vi "Dynamixel Single Function.vi"(6 "data":u32, 7 "Function":T1, 10 "dynamixel_id":u8=1, 11 "Com port":refnum<visa-resource-name> caption="instrument handle") -> (0 "error out":errorcluster, 1 "function return":i32)   [LabVIEW 2022 SP3]
uses:
  Sub Vis/Dynamixel Commands.ctl
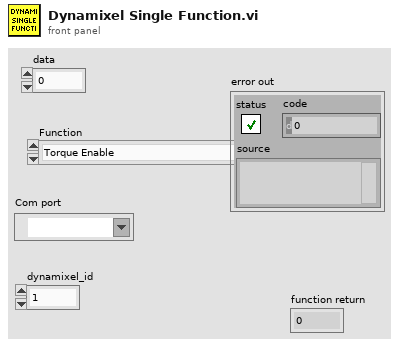
[diagram p1: front panel]
types:
  T1 = typedef "Dynamixel Commands.ctl" = enum16{"Torque Enable", "Present Position", "Threshold", "Max Position Limit", "Acceleration Profile", "Velocity Profile", "Goal Position", "Position Proportional Gain", "Position Integral Gain", "Position Differential Gain ", "Shutdown", "Write Operating Mode", "Read Operating Mode"}
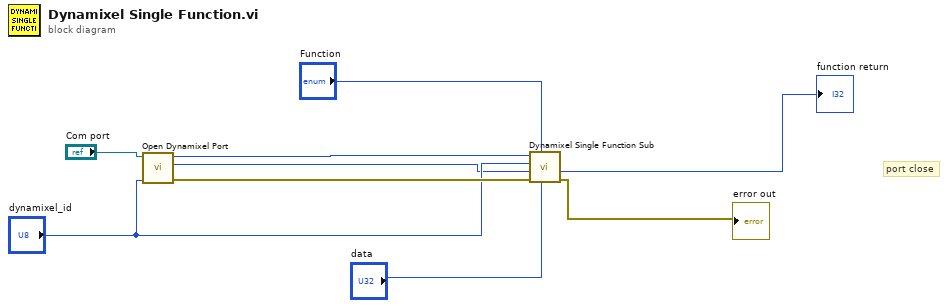
[diagram p0: block diagram]
diagram:
  # "port close"
  n1 = call "Open Dynamixel Port.vi"("dynamixel_id"="dynamixel_id", "Com port"="Com port") -> ("error out"=w6:errorcluster, "Model Number"=w1:u32, "port_num"=w5:i32)  [unwired: 7 in]
  n2 = call "Dynamixel Single Function Sub.vi"("data"="data", "Function"="Function", "error In"=w6, "Model Number"=w1, "dynamixel_id"="dynamixel_id", "port_num"=w5) -> ("error out"=→"error out":errorcluster, "function return"=→"function return":i32)  [unwired: 4 in]
